vi "Check Reference.vi"(8 "error in (no error)":errorcluster, 10 "Cluster in":refnum<vi>, 11 "SSL UDP Receiver 3":T1) -> (0 "error out":errorcluster, 3 "SSL UDP Receiver":T1)   [LabVIEW 2018]
uses:
  Control/SSL UDP Address.ctl
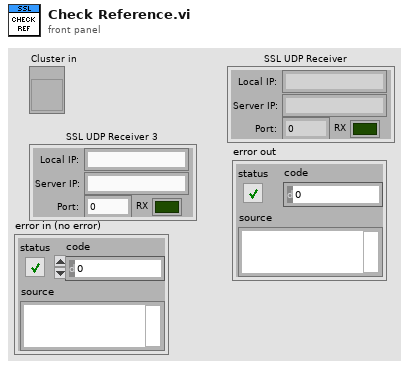
[diagram p1: front panel]
types:
  T1 = typedef "SSL UDP Address.ctl" = cluster{"Port:":u16, "Server IP:":string, "Local IP:":string, "RX":bool}
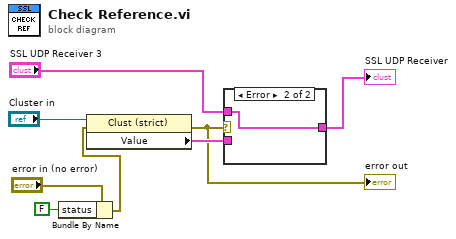
[diagram p0: block diagram]
diagram:
  n1 = Bundle By Name(cluster="error in (no error)", "status"=FALSE) -> (w1:errorcluster)
  n2 = property on="Property Node" class="Clust (strict)"(reference="Cluster in", error in=w1) -> (error out=w4:errorcluster, "Value"=w6:T1)  [unwired: 1 out]
  "error out" <- w4
  n3 = case shown="Error" w4 {
    tunnel: "SSL UDP Receiver 3" -> [_ w10]
    tunnel: w6 -> [w9 _]
    tunnel: [w9 w10] -> w7
    frame No Error {
    }
    frame Error {
    }
  }
  "SSL UDP Receiver" <- w7
